vi "Global_CMD.vi"() -> ()   [LabVIEW 2016, in "TemplateSensor.lvlib"]
uses:
  TemplateSensor.lvlib
panel:
  in  "CMD_Template_DBL":dbl
  in  "CMD_Template_Bool":bool
  # "The Names of the Data items in the Global Variable MUST describe who the Single Writer is\nNaming Convention for Command Globals is:   \n\nCMD_SubSystem_Data Name\nExample:\nCMD_Drive_Mode\nCMD_Hopper_Fire Ball"
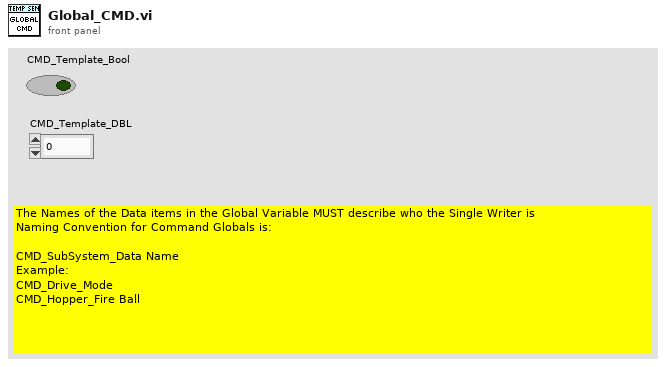
[diagram p1: front panel]
diagram:
